vi "Sort 2D Array (Numeric).vi"(10 "Sort by Cols":i32[](array[numeric]), 11 "Input Array":dbl[][](array[numeric])) -> (3 "Output Array":dbl[][](array[numeric]))   [LabVIEW 2010]
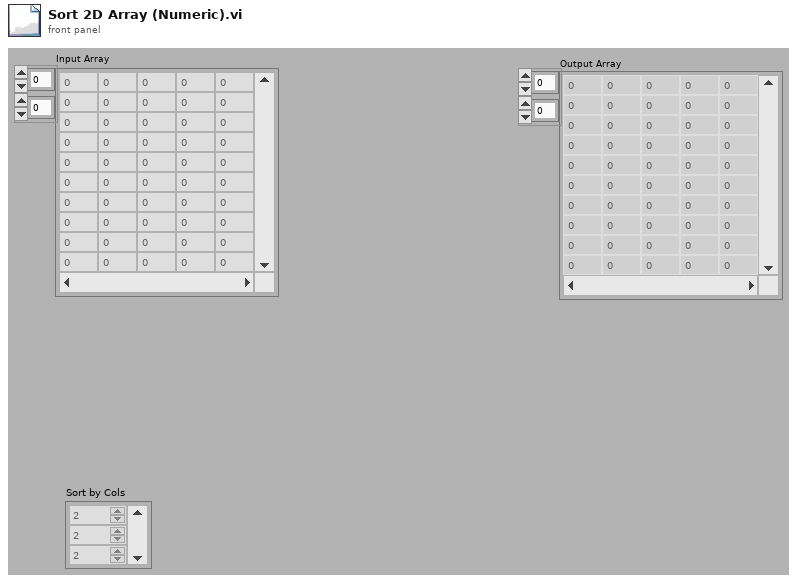
[diagram p1: front panel]
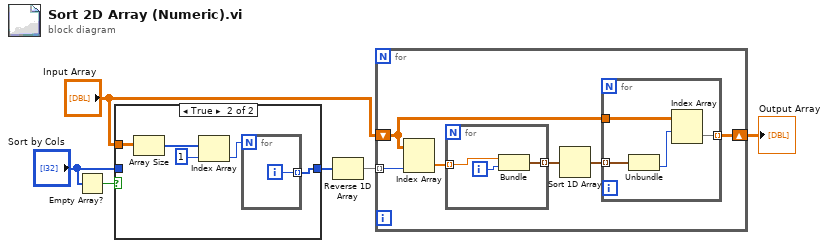
[diagram p0: block diagram]
diagram:
  n1 = Empty Array?(array="Sort by Cols") -> (empty?=w4:bool)
  n2 = case shown="True" w4 {
    tunnel: [w7 w8] -> w2
    tunnel: "Sort by Cols" -> [w7 _]
    tunnel: "Input Array" -> [_ w12]
    frame False {
    }
    frame True {
      n3 = Array Size(array=w12) -> (size(s)=w11:i32[])
      n4 = Index Array(array=w11, index=1) -> (element=w9:i32)
      n5 = for {
        N: w9 -> [_]
        tunnel: [w13] -> w8 mode=indexing
        i -> [w13]
      }
    }
  }
  n6 = Reverse 1D Array(array=w2) -> (reversed array=w6:i32[])
  n7 = for {
    tunnel: w6 -> [w19] mode=indexing
    shift-right: [w17] -> w5
    shift-left: "Input Array" -> [w16]
    n8 = Index Array(array=w16, index (col)=w19) -> (element=w18:dbl[])  [unwired: 1 in]
    n9 = for {
      tunnel: w18 -> [w20] mode=indexing
      tunnel: [w21] -> w14 mode=indexing
      i -> [w22]
      n10 = Bundle("Numeric"=w20, w22) -> (w21:cluster{"Numeric":dbl, i32})  [unwired: 1 in]
    }
    n11 = Sort 1D Array(array=w14) -> (sorted array=w15:cluster{"Numeric":dbl, i32}[])
    n12 = for {
      tunnel: w15 -> [w26] mode=indexing
      tunnel: w16 -> [w25]
      tunnel: [w24] -> w17 mode=indexing
      n13 = Unbundle(w26) -> (w23:i32)  [unwired: 1 out]
      n14 = Index Array(array=w25, index (row)=w23) -> (element=w24:dbl[])  [unwired: 1 in]
    }
  }
  "Output Array" <- w5
